vi "Keyence.Cmd.TuneCheck.vi"(8 "error in (no error)":errorcluster, 9 "Timeout [ms] (1000)":i32=1000, 11 "connection ID":refnum<k5>) -> (0 "error out":errorcluster, 2 "Tune succeded":bool, 3 "connection ID out":refnum<k5>)   [LabVIEW 2015]
panel:
  out "response 2":string
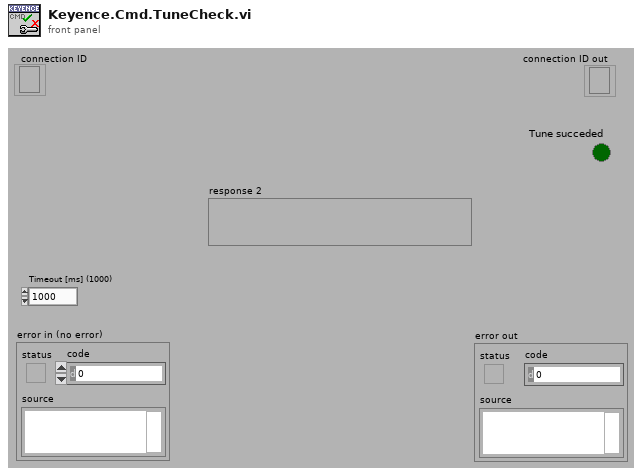
[diagram p1: front panel]
types:
  T1 = enum16{"Standard", "Buffered", "CRLF", "Immediate"}
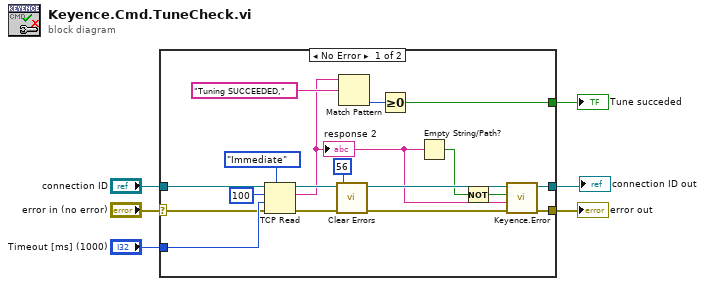
[diagram p0: block diagram]
diagram:
  n1 = case shown="No Error" "error in (no error)" {
    selector: "error in (no error)" -> [w11 w24]
    tunnel: [w10 w24] -> w6
    tunnel: "Timeout [ms] (1000)" -> [w22 _]
    tunnel: [w21 _] -> w3
    tunnel: "connection ID" -> [w20 w23]
    tunnel: [w19 w23] -> w1
    frame No Error {
      n2 = TCP Read(connection ID=w20, bytes to read=100, error in (no error)=w11, 7:T1."Immediate" ("mode (standard)"), 9:w22) -> (connection ID out=w19:refnum<k5>, data out=w7:string, error out=w15:errorcluster)
      "response 2" <- w7
      n3 = call <vilib>:"Clear Errors.vi"("error in (no error)"=w15, "specific error code to clear (0: all)"=56) -> ("error out"=w18:errorcluster)  [unwired: 4 in, 1 out]
      n4 = Match Pattern(string=w7, regular expression="Tuning SUCCEEDED,") -> (offset past match=w12:i32)  [unwired: 1 in, 3 out]
      n5 = Greater Or Equal To 0?(x=w12) -> (x >= 0?=w21:bool)
      n6 = Empty String/Path?(string/path=w7) -> (empty?=w8:bool)
      n7 = Not(x=w8) -> (.not. x?=w9:bool)
      n8 = call "Keyence.Error.vi"("error in (no error)"=w18, "Response"=w7, "Cmd ok"=w9) -> ("error out"=w10:errorcluster)  [unwired: 8 in]
    }
    frame Error {
    }
  }
  "error out" <- w6
  "Tune succeded" <- w3
  "connection ID out" <- w1
